vi "Nicht blockierende (Fehler) Meldung.vi"() -> ()   [LabVIEW 2015, in "SysLog.lvlib"]
doc: "Fehlermeldung zum Anzeigen der aktuellen Fehlermeldung und zum Durchblättern durch die gesammelten Fehlermeldungen. Zum Aufruf als Popup - liest die Fehlermeldungen aus dem zugehörigen FGV.\n#ErrLogHistory\nriw 8.6.2018"
uses:
  SysLog.lvlib
  Aktionen FGV SysLog.ctl
  Allgemein/allgemeine Sub-VIs.lvlib
panel:
  in  "Index":i32
  in  "Bildlaufleiste":i32(c297)
  out "Beschreibung":string
  out "Meldung":string
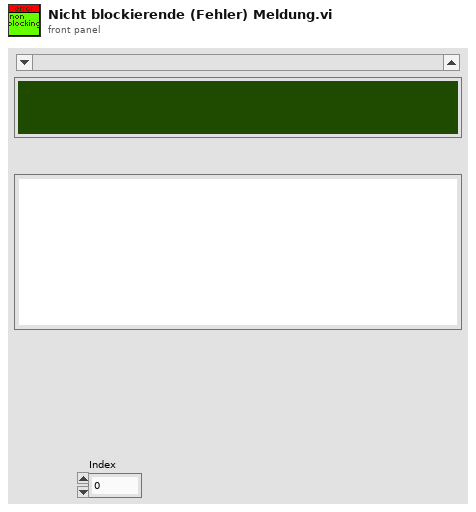
[diagram p1: front panel]
types:
  T1 = typedef "SysLog.lvlib/Aktionen FGV SysLog.ctl" = enum16{"initialisieren", "lesen", "schreiben", "history button ref"}
  T2 = cluster{"Anzeige Array":bool[], "Message Array":string[], "SysLog Incon Array":enum16{"OK", "Warnung", "Fehler"}[], "Status Message Array":string[], "Status SysLog Incon Array":enum16{"OK", "Warnung", "Fehler"}[]}
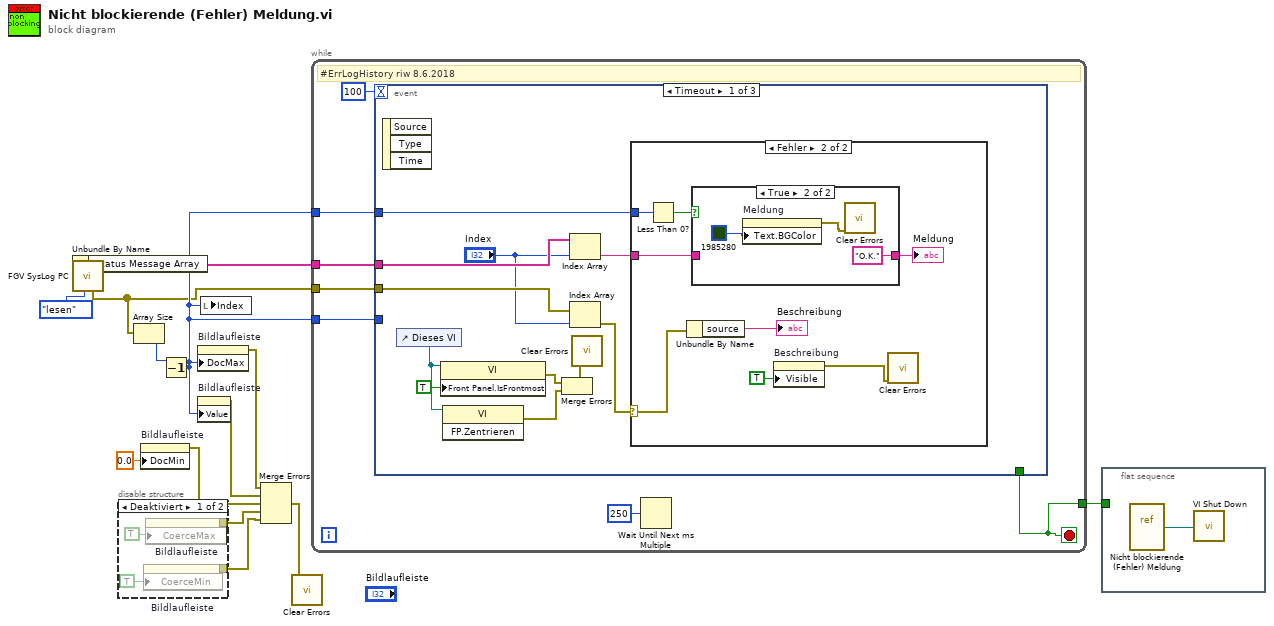
[diagram p0: block diagram]
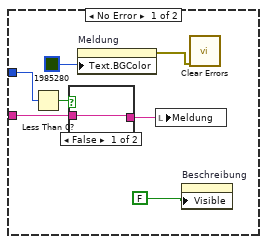
[diagram p3: hidden frame]
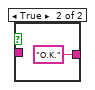
[diagram p4: hidden frame]
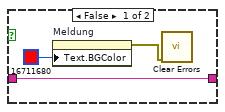
[diagram p5: hidden frame]
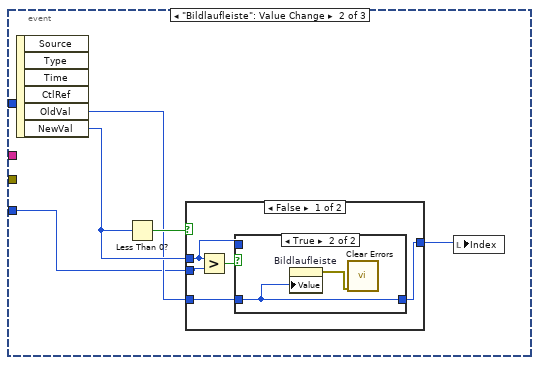
[diagram p6: hidden frame]
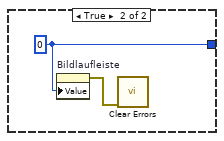
[diagram p8: hidden frame]
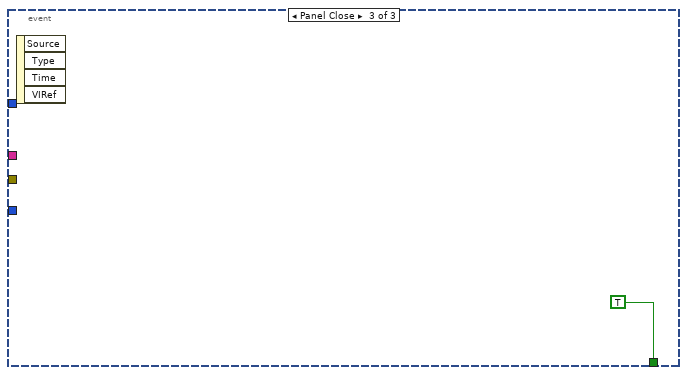
[diagram p9: hidden frame]
diagram:
  n1 = call "FGV SysLog PC.vi"("Aktion"=Aktionen_FGV_SysLog."lesen") -> ("Anzeige Cluster"=w3:T2, "Fehler out"=w2:errorcluster[])  [unwired: 7 in, 2 out]
  n2 = Unbundle By Name(w3) -> ("Status Message Array"=w1:string[])
  n3 = disable-structure shown="Deaktiviert" {
    disable-tunnel: [w16 _] -> w10
    disable-tunnel: [w15 _] -> w9
    frame Disabled {
      n4 = property on="Bildlaufleiste" class="Bildlauf (strikt)"("CoerceMin"=TRUE ("Auf Mindestwert setzen")) -> (error out=w15:errorcluster)  [unwired: 2 in, 1 out]
      n5 = property on="Bildlaufleiste" class="Bildlauf (strikt)"("CoerceMax"=TRUE ("Auf Höchstwert setzen")) -> (error out=w16:errorcluster)  [unwired: 2 in, 1 out]
    }
    frame Enabled {
    }
  }
  n6 = Array Size(array=w2) -> (size(s)=w13:i32)
  n7 = property on="Bildlaufleiste" class="Bildlauf (strikt)"("DocMin"=0.0 ("Dok Min")) -> (error out=w5:errorcluster)  [unwired: 2 in, 1 out]
  n8 = Decrement(x=w13) -> (x-1=w4:i32)
  n9 = property on="Bildlaufleiste" class="Bildlauf (strikt)"("DocMax"=w4) -> (error out=w7:errorcluster)  [unwired: 2 in, 1 out]
  n10 = property on="Bildlaufleiste" class="Bildlauf (strikt)"("Value"=w4) -> (error out=w6:errorcluster)  [unwired: 2 in, 1 out]
  n11 = local write "Index"(w4) -> ()
  n12 = Merge Errors(w7, w6, w5, w10, w9) -> (w11:errorcluster)
  n13 = call <vilib>:"Clear Errors.vi"("error in (no error)"=w11) -> ()  [unwired: 5 in, 2 out]
  n14 = while {
    tunnel: [w24] -> w14
    tunnel: w1 -> [w23]
    tunnel: w2 -> [w22]
    tunnel: w4 -> [w21]
    tunnel: w4 -> [w20]
    stop <- w24 stop-if-true
    # "#ErrLogHistory riw 8.6.2018"
    n15 = event shown="[0] Timeout" {
      selector: _ -> [_ _ _]
      dyn-events: _ -> [_ _ _]
      timeout: 100 -> [_ _ _]
      tunnel: w23 -> [w34 _ _]
      tunnel: w22 -> [w33 _ _]
      tunnel: [_ _ TRUE] -> w24
      tunnel: w21 -> [w26 _ _]
      tunnel: w20 -> [_ w60 _]
      event Timeout {
        n16 = event-data() -> ()  [unwired: 1 in, 3 out]
        n17 = control-ref of="Dieses VI"() -> (w29:refnum<vi>)
        n18 = property class="VI"(reference=w29, "Front Panel.IsFrontmost"=TRUE ("Frontpanel-Fenster:Ist im Vordergrund")) -> (error out=w30:errorcluster)  [unwired: 1 in, 1 out]
        n19 = invoke class="VI" method="FP.Zentrieren"(reference=w29) -> (error out=w27:errorcluster)  [unwired: 2 in, 2 out]
        n20 = Merge Errors(w30, w27) -> (w28:errorcluster)
        n21 = Index Array(array=w34, index="Index") -> (element=w36:string)
        n22 = Index Array(array=w33, index="Index") -> (element=w35:errorcluster)
        n23 = call <vilib>:"Clear Errors.vi"("error in (no error)"=w28) -> ()  [unwired: 5 in, 2 out]
        n24 = case shown="Fehler" w35 {
          selector: w35 -> [_ w53]
          tunnel: w36 -> [w38 w47]
          tunnel: w26 -> [w40 w49]
          frame No Error {
            n25 = Less Than 0?(x=w40) -> (x < 0?=w39:bool)
            n26 = case shown="False" w39 {
              tunnel: w38 -> [w44 _]
              tunnel: [w44 "O.K." ("String")] -> w37
              frame False {
              }
              frame True {
              }
            }
            n27 = property on="Meldung" class="Str"("Text.BGColor"=u32 1985280) -> (error out=w42:errorcluster)  [unwired: 2 in, 1 out]
            n28 = local write "Meldung"(w37) -> ()
            n29 = property on="Beschreibung" class="Str"("Visible"=FALSE ("Sichtbar")) -> ()  [unwired: 2 in, 2 out]
            n30 = call <vilib>:"Clear Errors.vi"("error in (no error)"=w42) -> ()  [unwired: 5 in, 2 out]
          }
          frame Error {
            n31 = Less Than 0?(x=w49) -> (x < 0?=w48:bool)
            n32 = Unbundle By Name(w53) -> ("source"=→"Beschreibung":string)
            n33 = case shown="True" w48 {
              tunnel: w47 -> [w56 _]
              tunnel: [w56 "O.K." ("String")] -> w46
              frame False {
                n34 = property on="Meldung" class="Str"("Text.BGColor"=u32 16711680) -> (error out=w55:errorcluster)  [unwired: 2 in, 1 out]
                n35 = call <vilib>:"Clear Errors.vi"("error in (no error)"=w55) -> ()  [unwired: 5 in, 2 out]
              }
              frame True {
                n36 = property on="Meldung" class="Str"("Text.BGColor"=u32 1985280) -> (error out=w58:errorcluster)  [unwired: 2 in, 1 out]
                n37 = call <vilib>:"Clear Errors.vi"("error in (no error)"=w58) -> ()  [unwired: 5 in, 2 out]
              }
            }
            "Meldung" <- w46
            n38 = property on="Beschreibung" class="Str"("Visible"=TRUE ("Sichtbar")) -> (error out=w50:errorcluster)  [unwired: 2 in, 1 out]
            n39 = call <vilib>:"Clear Errors.vi"("error in (no error)"=w50) -> ()  [unwired: 5 in, 2 out]
          }
        }
      }
      event "Bildlaufleiste": Value Change {
        n40 = event-data() -> ("OldVal"=w61:i32, "NewVal"=w63:i32)  [unwired: 1 in, 4 out]
        n41 = Less Than 0?(x=w63) -> (x < 0?=w64:bool)
        n42 = case shown="False" w64 {
          tunnel: [w68 w74] -> w62
          tunnel: w63 -> [w66 _]
          tunnel: w61 -> [w67 _]
          tunnel: w60 -> [w65 _]
          frame False {
            n43 = Greater?(x=w66, y=w65) -> (0:w69:bool)
            n44 = case shown="True" w69 {
              tunnel: [w70 w72] -> w68
              tunnel: w67 -> [_ w72]
              tunnel: w66 -> [w70 _]
              frame False {
              }
              frame True {
                n45 = property on="Bildlaufleiste" class="Bildlauf (strikt)"("Value"=w72) -> (error out=w71:errorcluster)  [unwired: 2 in, 1 out]
                n46 = call <vilib>:"Clear Errors.vi"("error in (no error)"=w71) -> ()  [unwired: 5 in, 2 out]
              }
            }
          }
          frame True {
            w74 = 0
            n47 = property on="Bildlaufleiste" class="Bildlauf (strikt)"("Value"=w74) -> (error out=w73:errorcluster)  [unwired: 2 in, 1 out]
            n48 = call <vilib>:"Clear Errors.vi"("error in (no error)"=w73) -> ()  [unwired: 5 in, 2 out]
          }
        }
        n49 = local write "Index"(w62) -> ()
      }
      event Panel Close {
        n50 = event-data() -> ()  [unwired: 1 in, 4 out]
      }
    }
    n51 = Wait Until Next ms Multiple(millisecond multiple=u32 250 ("ms")) -> ()  [unwired: 1 out]
  }
  n52 = flat-sequence {
    tunnel: w14 -> [_]
    frame #0 {
      n53 = vi-ref "Nicht blockierende (Fehler) Meldung.vi"() -> (w76:refnum<vi>)
      n54 = call "VI Shut Down.vi"("VI Referenz"=w76) -> ()  [unwired: 11 in]
    }
  }
